vi "chipKIT DP32.vi"() -> (0 "chipKIT DP32":T1={"DI Channels"=[0, 1, 2, 3, 4, 5, 6, 7, 8, 9, 10, 11, 12, 13, 14, 15, 16, 17, 18], "DO Channels"=[0, 1, 2, 3, 4, 5, 6, 7, 8, 9, 10, 11, 12, 13, 14, 15, 16, 17, 18], "AI"=[0, 1, 2, 3, 4, 5, 6, 7, 8], "AO"=[], "PWM"=[2, 3, 6, 8, 13], "QE"=[], "UART"=[0, 1], "I2C 2"=[1], "SPI"=[0], "CAN"=[], "AI Ref (V)"=3.3, "Firmware Program Interfaces"=[enum."Serial / USB"], "Firmware Versions"=[{"Name"="LINX chipKIT DP32 Serial/USB", "Relative Path"="\\Digilent\\chipKIT\\DP32\\DP32_Serial_USB_Debug.hex ", "Firmware Interface"=enum."Serial "}], "Name"="chipKIT DP32", "AO Resolution (Bits)"=0, "AO Ref (V)"=0.0})   [LabVIEW 2013, in "LVH-LINX.lvlib"]
doc: "I/O description of the chipKIT DP32."
uses:
  <vilib>/LabVIEW Hacker/LINX/LVH-LINX.lvlib
  <vilib>/LabVIEW Hacker/LINX/Private/Type Defs/Devices/Generic Device.ctl
  <vilib>/LabVIEW Hacker/LINX/Private/Type Defs/Firmware Version.ctl
  <vilib>/LabVIEW Hacker/LINX/Private/Device/Type Defs/Firmware Interface.ctl
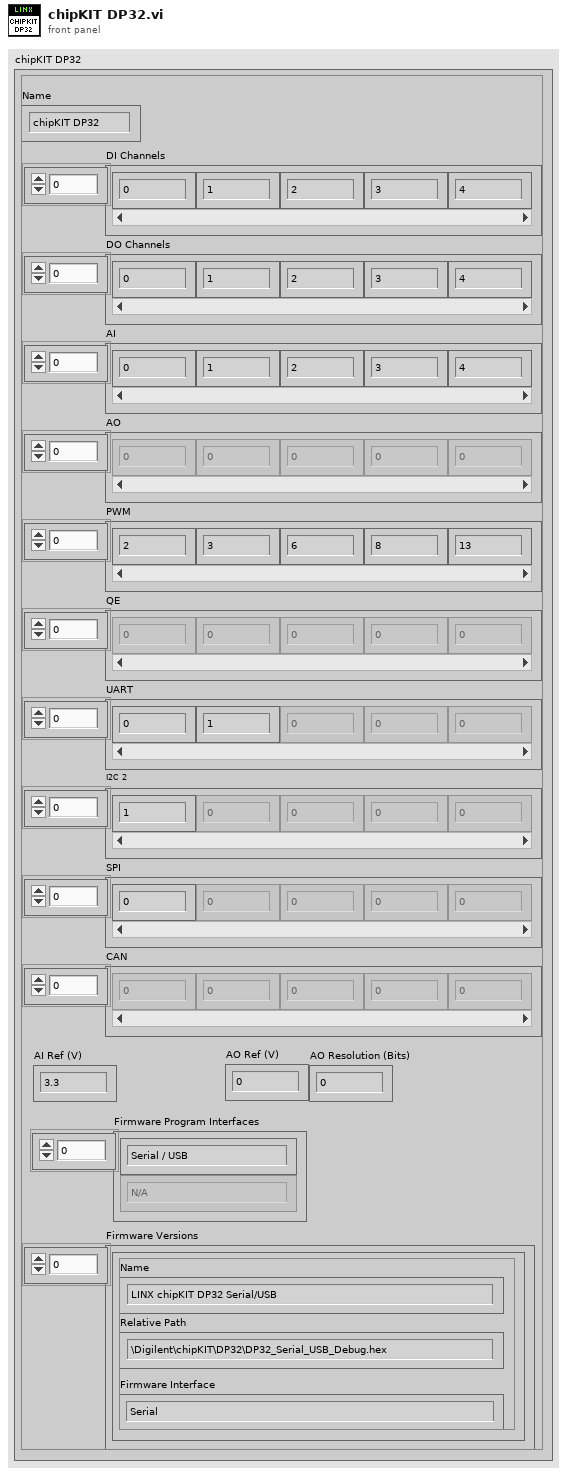
[diagram p1: front panel]
types:
  T1 = typedef "LVH-LINX.lvlib/Generic Device.ctl" = cluster{"DI Channels":u8[], "DO Channels":u8[], "AI":u8[], "AO":u8[], "PWM":u8[], "QE":u8[], "UART":u8[], "I2C 2":u8[], "SPI":u8[], "CAN":u8[], "AI Ref (V)":dbl, "Firmware Program Interfaces":enum16{"N/A", "Serial / USB", "USB", "TCP"}[], "Firmware Versions":T2[], "Name":string, "AO Resolution (Bits)":u8, "AO Ref (V)":dbl}
  T2 = typedef "LVH-LINX.lvlib/Firmware Version.ctl" = cluster{"Name":string, "Relative Path":string, "Firmware Interface":T3}
  T3 = typedef "LVH-LINX.lvlib/Firmware Interface.ctl" = enum32{"Serial ", "Ethernet", "WIFI"}
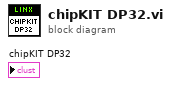
[diagram p0: block diagram]
diagram:
